vi "数据主动和反控发送.vi"() -> ()   [LabVIEW 2016, in "数据传输系统-06.lvlib"]
uses:
  <vilib>/ptbypt/NI_PtbyPt.lvlib
panel:
  out "QN":string
  out "队列中元素数量":i32
  out "元素":cluster{"命令编码CN":string, "QN":string}[](array[cluster])
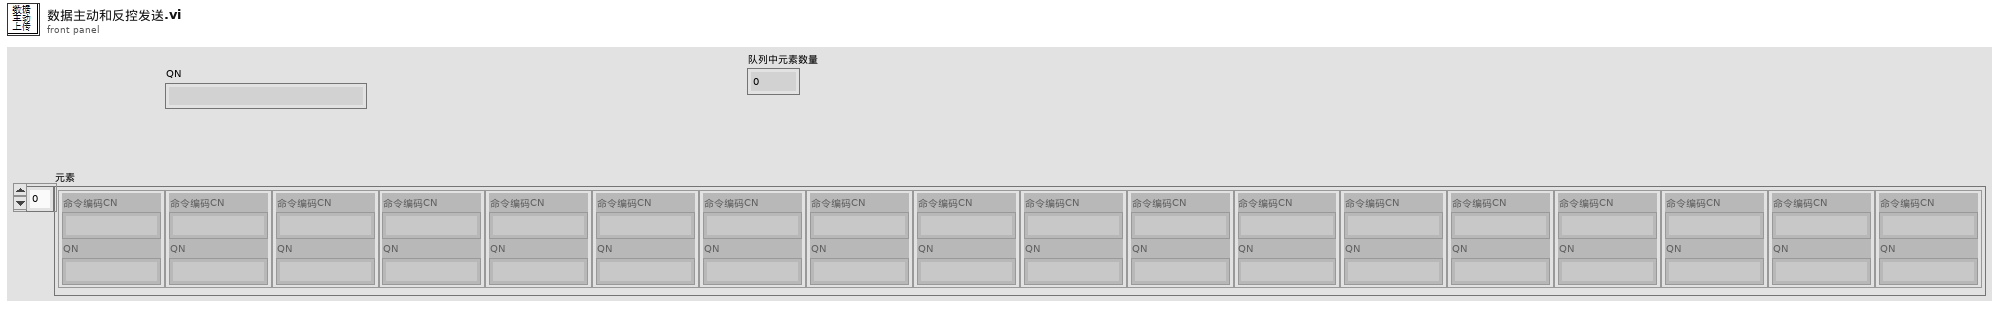
[diagram p1: front panel]
types:
  T1 = cluster{"setini":string, "sysini":string, "hechaini":string, "actualwrite":string, "actualread":string, "datasent":string, "反控命令信息队列":string, "反控与仪器交互":string}
  T2 = enum16{"00点", "01点", "02点", "03点", "04点", "05点", "06点", "07点", "08点", "09点", "10点", "11点", "12点", "13点", "14点", "15点", "16点", "17点", "18点", "19点", "20点", "21点", "22点", "23点"}
  T3 = enum16{"关闭", "星期日", "星期一", "星期二", "星期三", "星期四", "星期五", "星期六"}
  T4 = typedef "LVDateTimeRec.ctl" = cluster{"秒数的小数部分":dbl, "秒":i32, "分":i32, "时":i32, "日":i32, "月":i32, "年":i32, "天数（周）":i32, "天数（年）":i32, "DST":i32}
  T5 = cluster{"[0]":string, "[1]":string, "[2]":string, "[3]":string, "[4]":string, "[5]":string, "[6]":string, "[7]":string, "[8]":string, "[9]":string, "[10]":string, "[11]":string, "[12]":string, "[13]":string, "[14]":string, "[15]":string, "[16]":string, "[17]":string, "[18]":string, "[19]":string, "[20]":string, "[21]":string, "[22]":string, "[23]":string, "[24]":string, "[25]":string, "[26]":string, "[27]":string, "[28]":string, "[29]":string, "[30]":string, "[31]":string, "[32]":string, "[33]":string, "[34]":string, "[35]":string, "[36]":string}
  T6 = typedef "数据传输系统-06.lvlib/应用环境.ctl" = enum16{"STD", "GB212", "婉仪平台"}
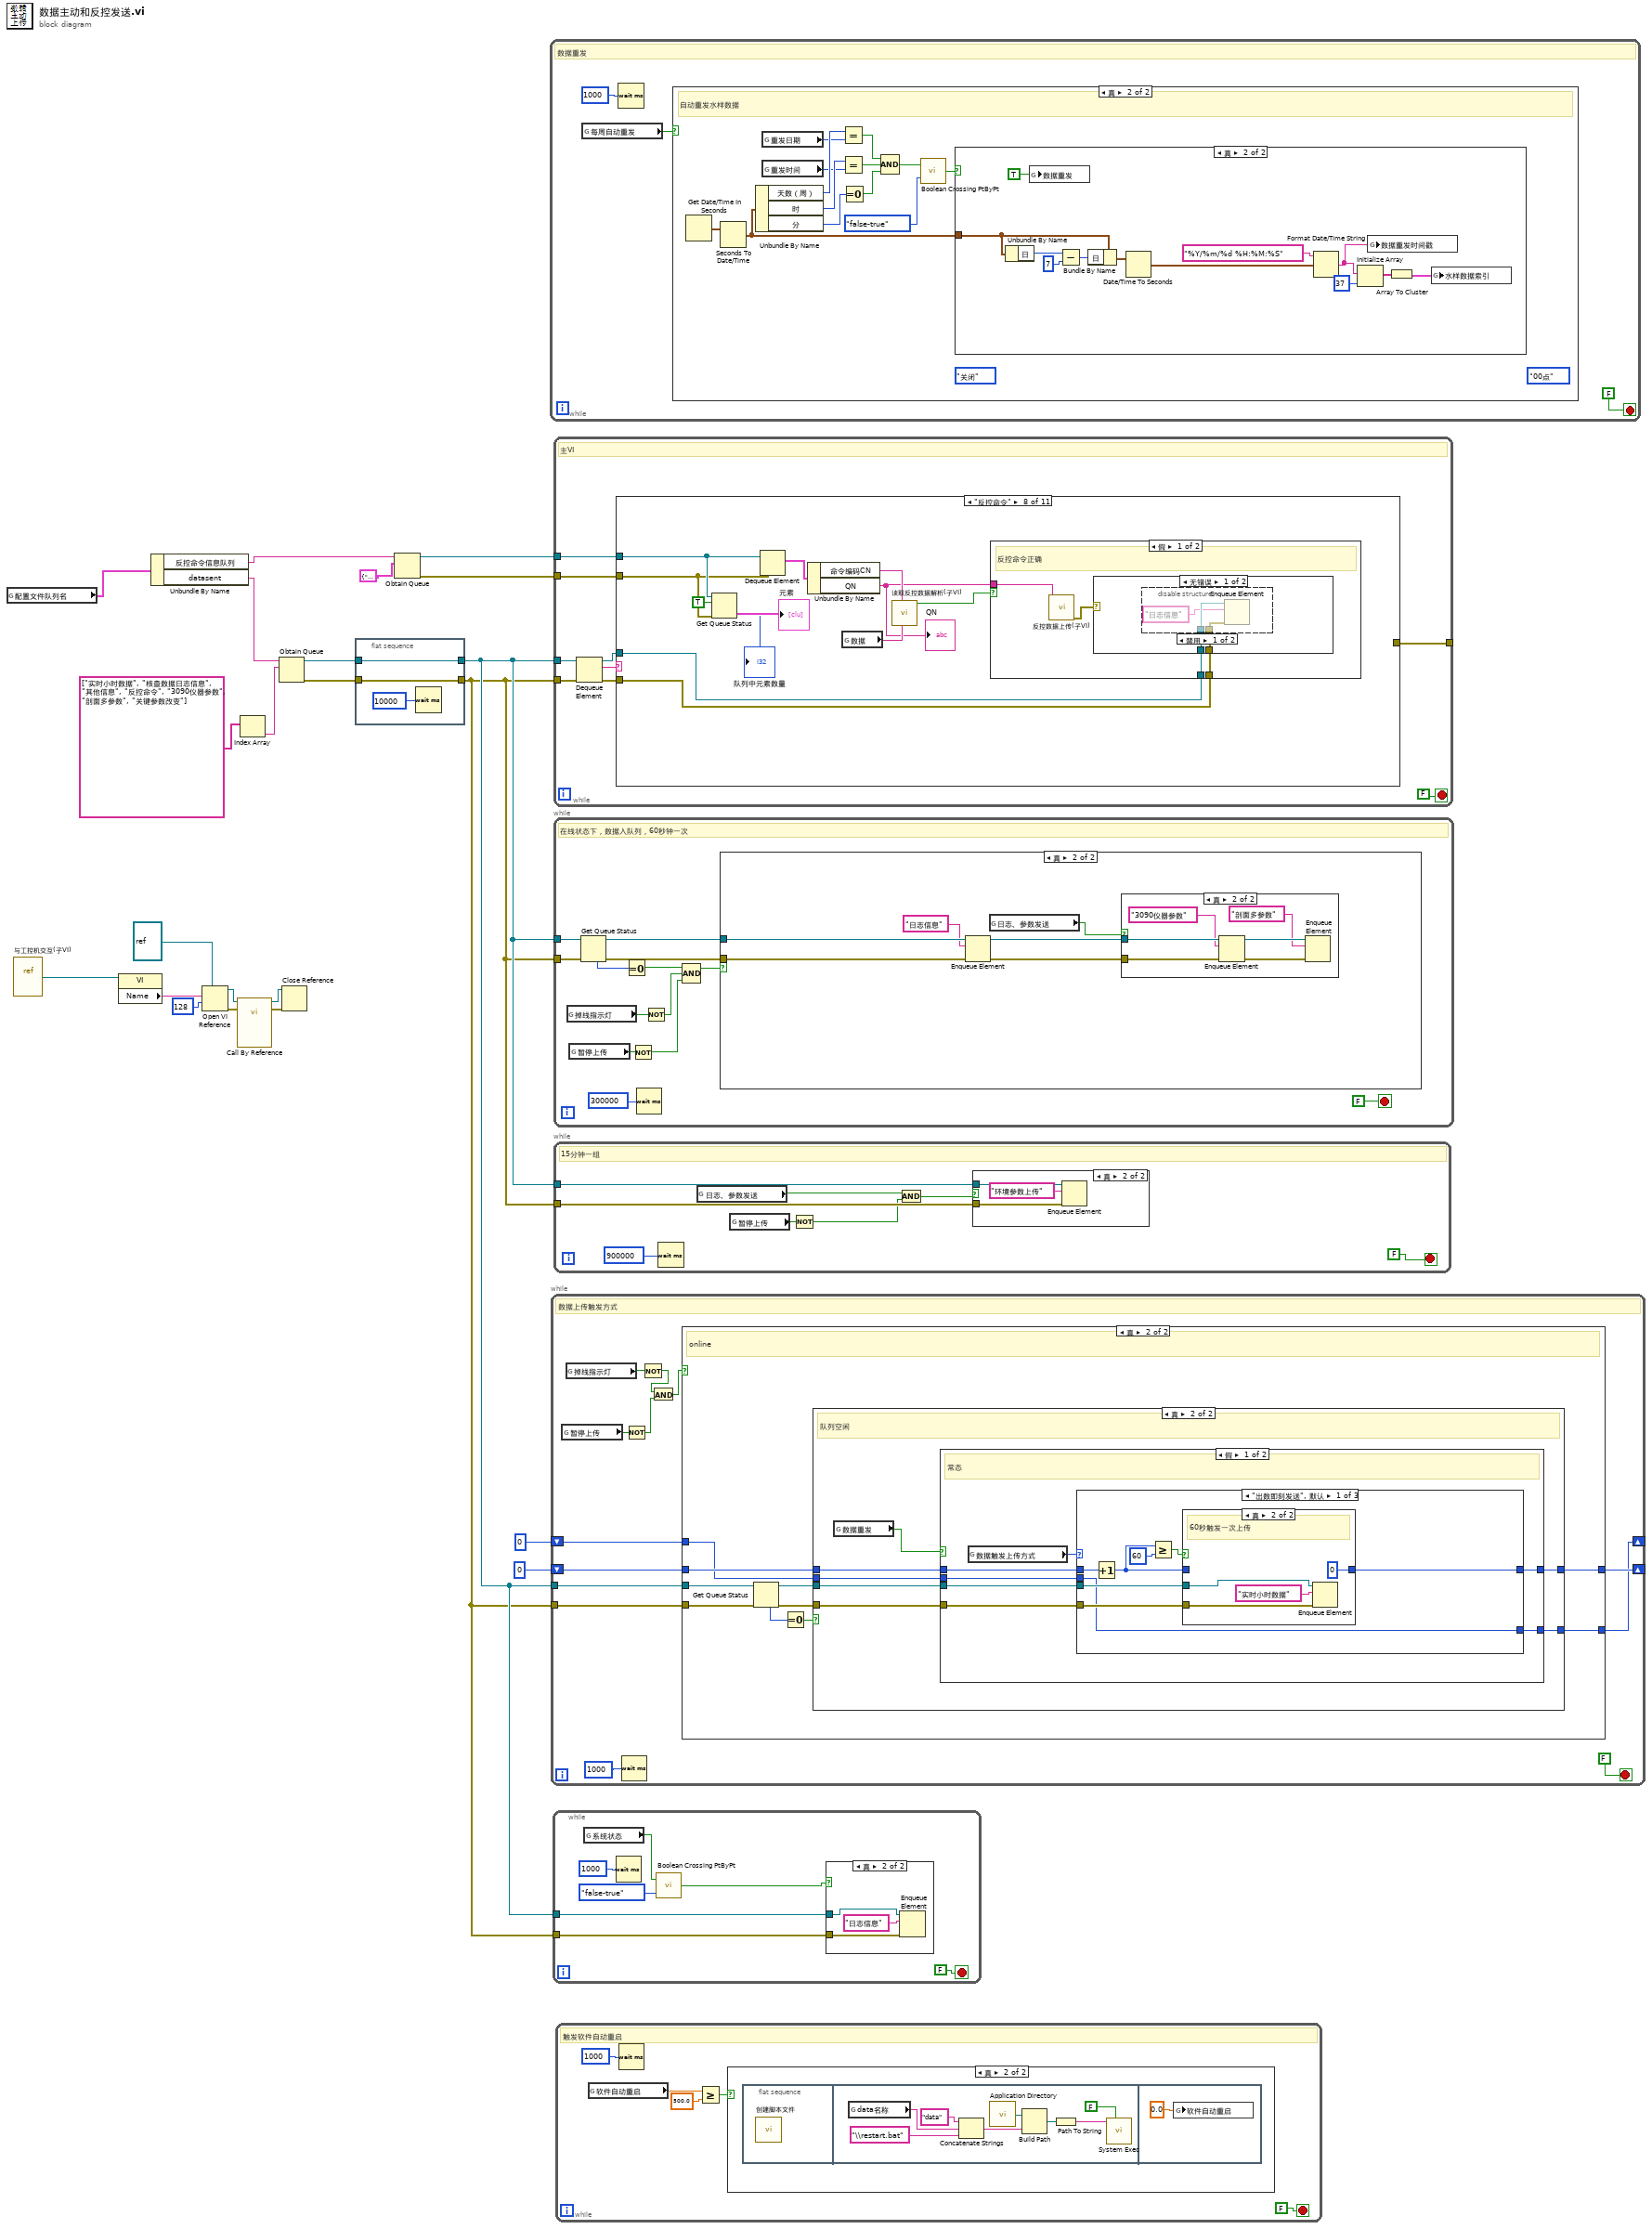
[diagram p0: block diagram]
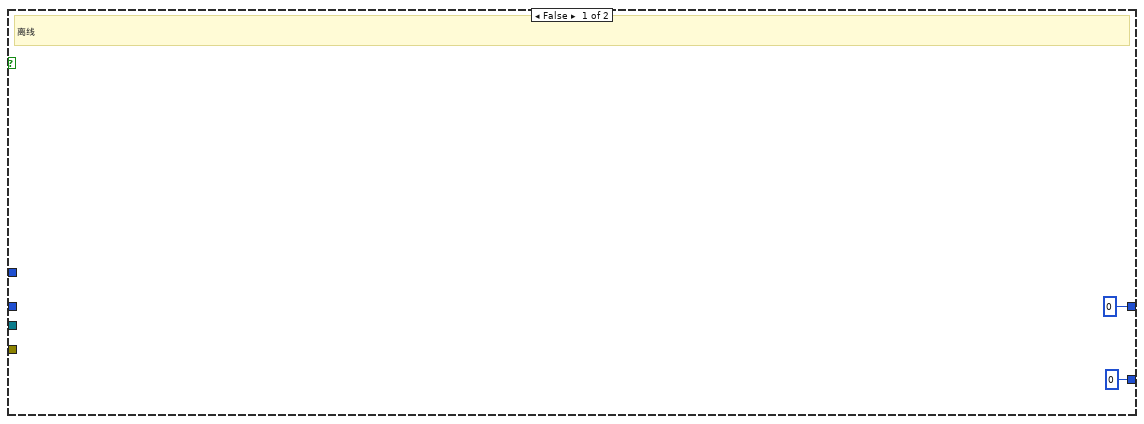
[diagram p4: hidden frame]
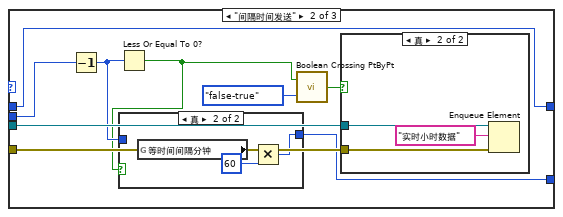
[diagram p7: hidden frame]
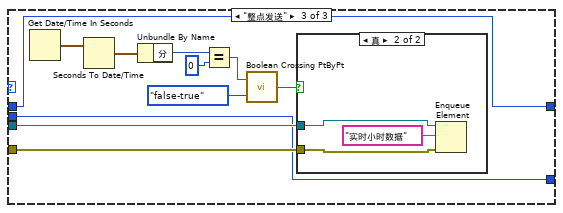
[diagram p10: hidden frame]
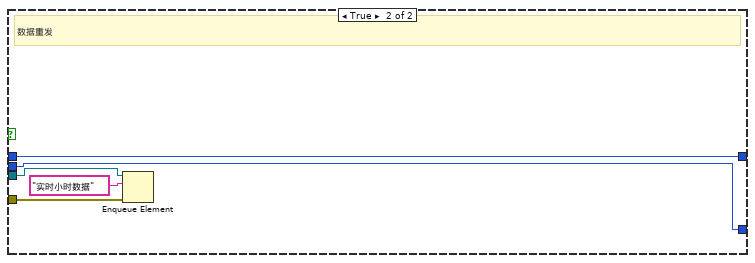
[diagram p12: hidden frame]
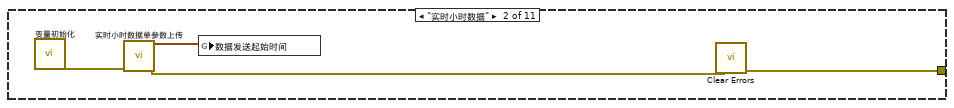
[diagram p19: hidden frame]
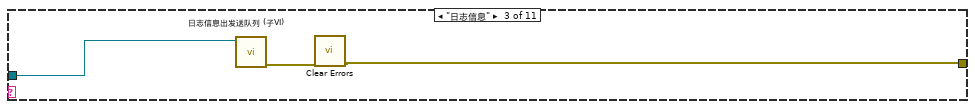
[diagram p20: hidden frame]
diagram:
  n1 = global read "全局1.vi" "配置文件队列名"() -> (w1:T1)
  n2 = vi-ref "与工控机交互(子VI).vi"() -> (w15:refnum<vi>)
  n3 = property class="VI"(reference=w15) -> ("Name"=w14:string)  [unwired: 1 in, 2 out]
  n4 = Unbundle By Name(w1) -> ("反控命令信息队列"=w5:string, "datasent"=w4:string)
  n5 = Open VI Reference(type specifier VI Refnum (for type only)=refnum<vi> refnum, vi path=w14, options=128 ("选项")) -> (vi reference=w12:refnum<vi>, error out=w2:errorcluster)  [unwired: 3 in]
  n6 = call-by-ref "?"(reference=w12, error in=w2) -> (reference out=w10:refnum<vi>, error out=w3:errorcluster)  [unwired: 12 in]
  n7 = Index Array(array=string[] ["实时小时数据", "核查数据日志信息", "其他信息", "反控命令", "3090仪器参数", "剖面多参数", "关键参数改变"]) -> (element=w16:string)  [unwired: 1 in]
  n8 = Obtain Queue(name (unnamed)=w4, element data type=w16) -> (queue out=w22:refnum<queue>, error out=w21:errorcluster)  [unwired: 3 in, 1 out]
  n9 = Close Reference(reference=w10, error in (no error)=w3) -> ()  [unwired: 1 out]
  n10 = flat-sequence {
    tunnel: w22 -> [w24]
    tunnel: [w24] -> w7
    tunnel: w21 -> [w23]
    tunnel: [w23] -> w6
    frame #0 {
      n11 = Wait (ms)(milliseconds to wait=u32 10000 ("等待时间（毫秒）")) -> ()  [unwired: 1 out]
    }
  }
  n12 = Obtain Queue(name (unnamed)=w5, element data type=cluster{"命令编码CN":string, "QN":string} {"命令编码CN"="", "QN"=""}) -> (queue out=w19:refnum<queue>, error out=w18:errorcluster)  [unwired: 3 in, 1 out]
  n13 = while {
    stop <- FALSE stop-if-true
    # "数据重发"
    n14 = global read "断电保存全局.vi" "每周自动重发"() -> (w27:bool)
    n15 = Wait (ms)(milliseconds to wait=u32 1000 ("等待时间（毫秒）")) -> ()  [unwired: 1 out]
    n16 = case shown="真" w27 {
      frame False {
      }
      frame True {
        (unwired) T2."00点"
        (unwired) T3."关闭"
        # "自动重发水样数据"
        n17 = Get Date/Time In Seconds() -> (seconds since 1Jan1904=w41:timestamp)
        n18 = Seconds To Date/Time(time stamp (now)=w41) -> (date time rec=w35:T4)  [unwired: 1 in]
        n19 = Unbundle By Name(w35) -> ("天数（周）"=w40:i32, "时"=w31:i32, "分"=w39:i32)
        n20 = global read "断电保存全局.vi" "重发日期"() -> (w30:T3)
        n21 = global read "断电保存全局.vi" "重发时间"() -> (w29:T2)
        n22 = Equal?(x=w40, y=w30) -> (x = y?=w38:bool)
        n23 = Equal?(x=w31, y=w29) -> (x = y?=w37:bool)
        n24 = Equal To 0?(x=w39) -> (x = 0?=w36:bool)
        n25 = Compound Arithmetic op=AND ("复合运算")(w38, w37, w36) -> (w34:bool)
        n26 = call <vilib>:"Boolean Crossing PtByPt.vi"("direction"=enum16{"either", "false-true", "true-false"}."false-true", "input"=w34) -> ("crossing"=w33:bool)  [unwired: 1 in]
        n27 = case shown="真" w33 {
          tunnel: w35 -> [_ w49]
          frame False {
          }
          frame True {
            n28 = Unbundle By Name(w49) -> ("日"=w52:i32)
            n29 = global write "断电保存全局.vi" "数据重发"(TRUE ("数据重发")) -> ()
            n30 = Subtract(x=w52, y=7) -> (x-y=w50:i32)
            n31 = Bundle By Name(cluster=w49, "日"=w50) -> (w53:T4)
            n32 = Date/Time To Seconds(2:w53) -> (0:w48:timestamp)  [unwired: 1 in]
            n33 = Format Date/Time String(time format string (%c)="%Y/%m/%d %H:%M:%S" ("时间格式字符串(%c)"), seconds (now)=w48) -> (date/time string=w42:string)  [unwired: 1 in]
            n34 = Initialize Array(w42, 37 ("维数大小")) -> (w44:string[])
            n35 = global write "断电保存全局.vi" "数据重发时间戳"(w42) -> ()
            n36 = Array To Cluster(array=w44) -> (cluster=w43:T5)
            n37 = global write "全局 水样时间.vi" "水样数据索引"(w43) -> ()
          }
        }
      }
    }
  }
  n38 = while {
    tunnel: w7 -> [w61]
    tunnel: w6 -> [w60]
    shift-right: [w63] -> _
    shift-left: 0 -> [w64]
    shift-right: [w54] -> _
    shift-left: 0 -> [w55]
    stop <- FALSE stop-if-true
    # "数据上传触发方式"
    n39 = global read "断电保存全局.vi" "暂停上传"() -> (w58:bool)
    n40 = global read "全局 数据发送重叠.vi" "掉线指示灯"() -> (w65:bool)
    n41 = Wait (ms)(milliseconds to wait=u32 1000 ("等待时间（毫秒）")) -> ()  [unwired: 1 out]
    n42 = Not(x=w58) -> (.not. x?=w57:bool)
    n43 = Not(x=w65) -> (.not. x?=w59:bool)
    n44 = And(x=w59, y=w57) -> (x .and. y?=w56:bool)
    n45 = case shown="真" w56 {
      tunnel: w64 -> [_ w78]
      tunnel: [0 w77] -> w63
      tunnel: w61 -> [_ w75]
      tunnel: w60 -> [_ w74]
      tunnel: w55 -> [_ w70]
      tunnel: [0 w69] -> w54
      frame False {
        # "离线"
      }
      frame True {
        # "online"
        n46 = Get Queue Status(queue=w75, error in (no error)=w74) -> (queue out=w72:refnum<queue>, error out=w71:errorcluster, # elements in queue=w76:i32)  [unwired: 1 in, 5 out]
        n47 = Equal To 0?(x=w76) -> (x = 0?=w73:bool)
        n48 = case shown="真" w73 {
          tunnel: w72 -> [_ w87]
          tunnel: w71 -> [_ w86]
          tunnel: w78 -> [w80 w85]
          tunnel: [w80 w84] -> w77
          tunnel: w70 -> [w79 w83]
          tunnel: [w79 w82] -> w69
          frame False {
            # "队列忙碌中"
          }
          frame True {
            # "队列空闲"
            n49 = global read "断电保存全局.vi" "数据重发"() -> (w81:bool)
            n50 = case shown="假" w81 {
              tunnel: w87 -> [w94 w141]
              tunnel: w86 -> [w93 w140]
              tunnel: w85 -> [w91 w139]
              tunnel: [w90 w139] -> w84
              tunnel: w83 -> [w89 w138]
              tunnel: [w88 w138] -> w82
              frame False {
                # "常态"
                n51 = global read "断电保存全局.vi" "数据触发上传方式"() -> (w92:enum16{"出数即刻发送", "间隔时间发送", "整点发送"})
                n52 = case shown="\"出数即刻发送\", 默认" w92 {
                  tunnel: w94 -> [w97 w115 w128]
                  tunnel: w93 -> [w96 w114 w127]
                  tunnel: w91 -> [w102 w116 w126]
                  tunnel: [w98 w116 w126] -> w90
                  tunnel: w89 -> [w95 w111 w124]
                  tunnel: [w95 w110 w124] -> w88
                  frame "出数即刻发送", Default {
                    n53 = Increment(x=w102) -> (x+1=w99:i32)
                    n54 = Greater Or Equal?(x=w99, y=60) -> (x >= y?=w100:bool)
                    n55 = case shown="真" w100 {
                      tunnel: w99 -> [w103 _]
                      tunnel: [w103 0] -> w98
                      tunnel: w97 -> [_ w105]
                      tunnel: w96 -> [_ w104]
                      frame False {
                      }
                      frame True {
                        # "60秒触发一次上传"
                        n56 = Enqueue Element(queue=w105, element="实时小时数据" ("元素"), error in (no error)=w104) -> ()  [unwired: 1 in, 3 out]
                      }
                    }
                  }
                  frame "间隔时间发送" {
                    n57 = Decrement(x=w111) -> (x-1=w109:i32)
                    n58 = Less Or Equal To 0?(x=w109) -> (x <= 0?=w108:bool)
                    n59 = case shown="真" w108 {
                      tunnel: w109 -> [w117 _]
                      tunnel: [w117 w118] -> w110
                      frame False {
                      }
                      frame True {
                        n60 = global read "断电保存全局.vi" "等时间间隔分钟"() -> (w119:i32)
                        n61 = Multiply(x=w119, y=60) -> (x*y=w118:i32)
                      }
                    }
                    n62 = call <vilib>:"Boolean Crossing PtByPt.vi"("direction"=enum16{"either", "false-true", "true-false"}."false-true", "input"=w108) -> ("crossing"=w112:bool)  [unwired: 1 in]
                    n63 = case shown="真" w112 {
                      tunnel: w115 -> [_ w122]
                      tunnel: w114 -> [_ w121]
                      frame False {
                      }
                      frame True {
                        n64 = Enqueue Element(queue=w122, element="实时小时数据" ("元素"), error in (no error)=w121) -> ()  [unwired: 1 in, 3 out]
                      }
                    }
                  }
                  frame "整点发送" {
                    n65 = Get Date/Time In Seconds() -> (seconds since 1Jan1904=w133:timestamp)
                    n66 = Seconds To Date/Time(time stamp (now)=w133) -> (date time rec=w134:T4)  [unwired: 1 in]
                    n67 = Unbundle By Name(w134) -> ("分"=w132:i32)
                    n68 = Equal?(x=w132, y=0) -> (x = y?=w130:bool)
                    n69 = call <vilib>:"Boolean Crossing PtByPt.vi"("direction"=enum16{"either", "false-true", "true-false"}."false-true", "input"=w130) -> ("crossing"=w125:bool)  [unwired: 1 in]
                    n70 = case shown="真" w125 {
                      tunnel: w128 -> [_ w136]
                      tunnel: w127 -> [_ w135]
                      frame False {
                      }
                      frame True {
                        n71 = Enqueue Element(queue=w136, element="实时小时数据" ("元素"), error in (no error)=w135) -> ()  [unwired: 1 in, 3 out]
                      }
                    }
                  }
                }
              }
              frame True {
                # "数据重发"
                n72 = Enqueue Element(queue=w141, element="实时小时数据" ("元素"), error in (no error)=w140) -> ()  [unwired: 1 in, 3 out]
              }
            }
          }
        }
      }
    }
  }
  n73 = while {
    tunnel: w7 -> [w145]
    tunnel: w6 -> [w144]
    stop <- FALSE stop-if-true
    n74 = global read "全局1.vi" "系统状态"() -> (w147:bool)
    n75 = Wait (ms)(milliseconds to wait=u32 1000 ("等待时间（毫秒）")) -> ()  [unwired: 1 out]
    n76 = call <vilib>:"Boolean Crossing PtByPt.vi"("direction"=enum16{"either", "false-true", "true-false"}."false-true", "input"=w147) -> ("crossing"=w143:bool)  [unwired: 1 in]
    n77 = case shown="真" w143 {
      tunnel: w145 -> [_ w150]
      tunnel: w144 -> [_ w151]
      frame False {
      }
      frame True {
        n78 = Enqueue Element(queue=w150, element="日志信息" ("元素"), error in (no error)=w151) -> ()  [unwired: 1 in, 3 out]
      }
    }
  }
  n79 = while {
    tunnel: w7 -> [w155]
    tunnel: w6 -> [w154]
    tunnel: w19 -> [w157]
    tunnel: w18 -> [w156]
    tunnel: [w153] -> _
    stop <- FALSE stop-if-true
    # "主VI"
    n80 = Dequeue Element(queue=w155, error in (no error)=w154) -> (queue out=w159:refnum<queue>, element=w160:string, error out=w158:errorcluster)  [unwired: 1 in, 1 out]
    n81 = case shown="\"反控命令\"" w160 {
      tunnel: w159 -> [_ _ w166 _ _ _ _ w188 _ _ _]
      tunnel: w158 -> [_ _ _ _ _ _ _ w187 _ _ _]
      tunnel: w157 -> [_ _ _ _ _ _ _ w198 _ _ _]
      tunnel: w156 -> [_ _ _ _ _ _ _ w197 _ _ _]
      tunnel: [_ w164 w167 w174 w180 w185 _ _ w209 w215 w220] -> w153
      frame Default {
      }
      frame "实时小时数据" {
        n82 = call "变量初始化.vi"() -> ("错误输出"=w162:errorcluster)  [unwired: 11 in]
        n83 = call "实时小时数据单参数上传.vi"("错误输入（无错误）"=w162) -> ("数据发送起始时间"=w165:timestamp, "error out"=w163:errorcluster)  [unwired: 13 in]
        n84 = global write "全局1.vi" "数据发送起始时间"(w165) -> ()
        n85 = call <vilib>:"Clear Errors.vi"("error in (no error)"=w163) -> ("error out"=w164:errorcluster)  [unwired: 5 in, 1 out]
      }
      frame "日志信息" {
        n86 = call "日志信息出发送队列 (子VI).vi"("queue out"=w166) -> ("错误输出"=w168:errorcluster)  [unwired: 10 in]
        n87 = call <vilib>:"Clear Errors.vi"("error in (no error)"=w168) -> ("error out"=w167:errorcluster)  [unwired: 5 in, 1 out]
      }
      frame "关键参数改变" {
        n88 = global read "断电保存全局.vi" "仪器参数发送"() -> (w172:bool)
        n89 = global read "断电保存全局.vi" "应用环境"() -> (w173:T6)
        n90 = Equal?(x=w173, y=应用环境."STD" ("应用环境")) -> (x = y?=w171:bool)
        n91 = And(x=w172, y=w171) -> (x .and. y?=w170:bool)
        n92 = case shown="真" w170 {
          tunnel: [_ w175] -> w174
          frame False {
          }
          frame True {
            n93 = call "仪器参数改变发送 (子VI).vi"() -> ("错误输出"=w176:errorcluster)  [unwired: 11 in]
            n94 = call "采配水仪器参数改变发送 (子VI).vi"("错误输入"=w176) -> ("错误输出"=w175:errorcluster)  [unwired: 10 in]
          }
        }
      }
      frame "校准信息改变" {
        n95 = global read "断电保存全局.vi" "应用环境"() -> (w179:T6)
        n96 = Equal?(x=w179, y=应用环境."STD" ("应用环境")) -> (x = y?=w178:bool)
        n97 = case shown="真" w178 {
          tunnel: [_ w181] -> w180
          frame False {
          }
          frame True {
            n98 = call "校准信息改变发送 (子VI).vi"() -> ("错误输出"=w181:errorcluster)  [unwired: 11 in]
          }
        }
      }
      frame "3201告警信息改变" {
        n99 = global read "断电保存全局.vi" "应用环境"() -> (w184:T6)
        n100 = Equal?(x=w184, y=应用环境."婉仪平台") -> (x = y?=w183:bool)
        n101 = case shown="真" w183 {
          tunnel: [_ w186] -> w185
          frame False {
          }
          frame True {
            n102 = call "3201告警信息改变发送 (子VI).vi"() -> ("错误输出"=w186:errorcluster)  [unwired: 11 in]
          }
        }
      }
      frame "其他信息" {
      }
      frame "反控命令" {
        n103 = Get Queue Status(queue=w198, return elements? (F)=TRUE ("返回元素？(F)"), error in (no error)=w197) -> (# elements in queue=→"队列中元素数量":i32, elements=→"元素":cluster{"命令编码CN":string, "QN":string}[])  [unwired: 6 out]
        n104 = Dequeue Element(queue=w198, error in (no error)=w197) -> (element=w194:cluster{"命令编码CN":string, "QN":string})  [unwired: 1 in, 3 out]
        n105 = Unbundle By Name(w194) -> ("命令编码CN"=w193:string, "QN"=w192:string)
        "QN" <- w192
        n106 = global read "全局1.vi" "数据"() -> (w196:string)
        n107 = call "读取反控数据解析(子VI).vi"("数据"=w196, "命令编码CN"=w193) -> ("反控命令错误？"=w195:bool)  [unwired: 8 in, 1 out]
        n108 = case shown="假" w195 {
          tunnel: w192 -> [w202 _]
          tunnel: w188 -> [w200 _]
          tunnel: w187 -> [w199 _]
          frame False {
            # "反控命令正确"
            n109 = call "反控数据上传(子VI).vi"("QN"=w202) -> ("error out"=w201:errorcluster)  [unwired: 10 in]
            n110 = case shown="无错误" w201 {
              tunnel: w200 -> [w204 _]
              tunnel: w199 -> [w203 _]
              frame No Error {
                n111 = disable-structure shown="禁用" {
                  disable-tunnel: w204 -> [w207 _]
                  disable-tunnel: w203 -> [w206 _]
                  frame Disabled {
                    n112 = Enqueue Element(queue=w207, element="日志信息" ("元素"), error in (no error)=w206) -> ()  [unwired: 1 in, 3 out]
                  }
                  frame Enabled {
                  }
                }
              }
              frame Error {
              }
            }
          }
          frame True {
            # "反控命令错误"
          }
        }
      }
      frame "3090仪器参数" {
        n113 = global read "断电保存全局.vi" "应用环境"() -> (w208:T6)
        n114 = case shown="\"GB212\", 默认" w208 {
          tunnel: [w210 _] -> w209
          frame "STD" {
            n115 = call "3090仪器参数上传.vi"() -> ("error out"=w211:errorcluster)  [unwired: 15 in]
            n116 = call "变量初始化.vi"("错误输入（无错误）"=w211) -> ("错误输出"=w210:errorcluster)  [unwired: 10 in]
          }
          frame "GB212", Default {
          }
        }
      }
      frame "剖面多参数" {
        n117 = global read "断电保存全局.vi" "应用环境"() -> (w214:T6)
        n118 = call "剖面多参数上传.vi"() -> ("error out"=w213:errorcluster)  [unwired: 15 in]
        n119 = call <vilib>:"Clear Errors.vi"("error in (no error)"=w213) -> ("error out"=w212:errorcluster)  [unwired: 5 in, 1 out]
        n120 = case shown="\"GB212\", 默认" w214 {
          tunnel: [w217 w218] -> w215
          tunnel: w212 -> [w216 w218]
          frame "STD" {
            n121 = call "新剖面数据上传.vi"("错误输入（无错误）"=w216) -> ("error out"=w217:errorcluster)  [unwired: 14 in]
          }
          frame "GB212", Default {
            n122 = global write "断电保存全局.vi" "剖面数据重发"(FALSE ("剖面数据重发")) -> ()
          }
        }
      }
      frame "环境参数上传" {
        n123 = call "环境参数上传.vi"() -> ("error out"=w220:errorcluster)  [unwired: 15 in]
      }
    }
  }
  n124 = while {
    tunnel: w7 -> [w233]
    tunnel: w6 -> [w232]
    stop <- FALSE stop-if-true
    # "在线状态下，数据入队列，60秒钟一次"
    n125 = global read "全局 数据发送重叠.vi" "掉线指示灯"() -> (w226:bool)
    n126 = global read "断电保存全局.vi" "暂停上传"() -> (w222:bool)
    n127 = Get Queue Status(queue=w233, error in (no error)=w232) -> (queue out=w230:refnum<queue>, error out=w229:errorcluster, # elements in queue=w231:i32)  [unwired: 1 in, 5 out]
    n128 = Equal To 0?(x=w231) -> (x = 0?=w224:bool)
    n129 = Not(x=w222) -> (.not. x?=w221:bool)
    n130 = Wait (ms)(milliseconds to wait=u32 300000 ("等待时间（毫秒）")) -> ()  [unwired: 1 out]
    n131 = Not(x=w226) -> (.not. x?=w223:bool)
    n132 = Compound Arithmetic op=AND ("复合运算")(w224, w223, w221) -> (w225:bool)
    n133 = case shown="真" w225 {
      tunnel: w230 -> [_ w239]
      tunnel: w229 -> [_ w238]
      frame False {
      }
      frame True {
        n134 = Enqueue Element(queue=w239, element="日志信息" ("元素"), error in (no error)=w238) -> (queue out=w236:refnum<queue>, error out=w235:errorcluster)  [unwired: 1 in, 1 out]
        n135 = global read "断电保存全局.vi" "日志、参数发送"() -> (w234:bool)
        n136 = case shown="真" w234 {
          tunnel: w236 -> [_ w245]
          tunnel: w235 -> [_ w244]
          frame False {
          }
          frame True {
            n137 = Enqueue Element(queue=w245, element="3090仪器参数" ("元素"), error in (no error)=w244) -> (queue out=w242:refnum<queue>, error out=w241:errorcluster)  [unwired: 1 in, 1 out]
            n138 = Enqueue Element(queue=w242, element="剖面多参数" ("元素"), error in (no error)=w241) -> ()  [unwired: 1 in, 3 out]
          }
        }
      }
    }
  }
  n139 = while {
    tunnel: w7 -> [w251]
    tunnel: w6 -> [w250]
    stop <- FALSE stop-if-true
    # "15分钟一组"
    n140 = Wait (ms)(milliseconds to wait=u32 900000 ("等待时间（毫秒）")) -> ()  [unwired: 1 out]
    n141 = global read "断电保存全局.vi" "日志、参数发送"() -> (w248:bool)
    n142 = global read "断电保存全局.vi" "暂停上传"() -> (w249:bool)
    n143 = Not(x=w249) -> (.not. x?=w247:bool)
    n144 = And(x=w248, y=w247) -> (x .and. y?=w246:bool)
    n145 = case shown="真" w246 {
      tunnel: w251 -> [_ w255]
      tunnel: w250 -> [_ w254]
      frame False {
      }
      frame True {
        n146 = Enqueue Element(queue=w255, element="环境参数上传" ("元素"), error in (no error)=w254) -> ()  [unwired: 1 in, 3 out]
      }
    }
  }
  n147 = while {
    stop <- FALSE stop-if-true
    # "触发软件自动重启"
    n148 = global read "全局1.vi" "软件自动重启"() -> (w259:dbl)
    n149 = Wait (ms)(milliseconds to wait=u32 1000 ("等待时间（毫秒）")) -> ()  [unwired: 1 out]
    n150 = Greater Or Equal?(x=w259, y=500.0) -> (x >= y?=w257:bool)
    n151 = case shown="真" w257 {
      frame False {
      }
      frame True {
        n152 = flat-sequence {
          frame #0 {
            n153 = call "创建脚本文件.vi"() -> ()  [unwired: 11 in, 1 out]
          }
          frame #1 {
            n154 = global read "断电保存全局.vi" "data名称"() -> (w264:string)
            n155 = Concatenate Strings("data" ("名称或相对路径"), w264, "\\restart.bat" ("字符串")) -> (w262:string)
            n156 = call <vilib>:"Application Directory.vi"() -> ("Application Directory"=w268:path)
            n157 = Build Path(base path=w268, name or relative path=w262) -> (appended path=w269:path)
            n158 = Path To String(path=w269) -> (string=w266:string)
            n159 = call <vilib>:"System Exec.vi"("wait until completion? (T)"=FALSE, "command line"=w266) -> ()  [unwired: 6 in, 4 out]
          }
          frame #2 {
            n160 = global write "全局1.vi" "软件自动重启"(0.0 ("软件自动重启")) -> ()
          }
        }
      }
    }
  }
